vi "Get Serial Port Name.vi"(4 "Error In":errorcluster, 7 "PS Communication Port In":refnum<visa-resource-name>) -> (0 "Error Out":errorcluster, 2 "Serial Port Name":string, 3 "PS Communication Port Out":refnum<visa-resource-name>)   [LabVIEW 2024]
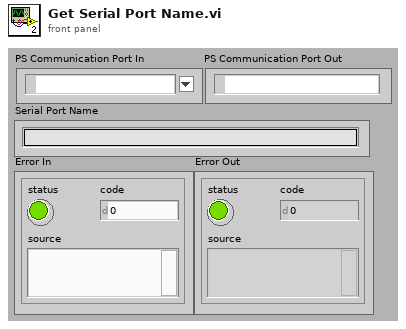
[diagram p1: front panel]
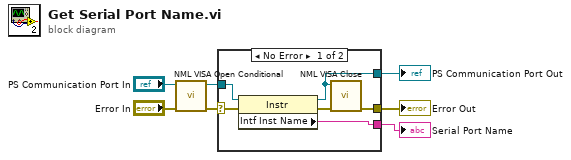
[diagram p0: block diagram]
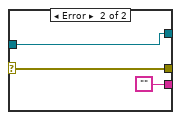
[diagram p2: hidden frame]
diagram:
  n1 = call "NML VISA Open Conditional.vi"("error in (no error)"="Error In", "VISA resource name"="PS Communication Port In") -> ("error out"=w5:errorcluster, "dup VISA Session"=w6:refnum<visa-resource-name>)  [unwired: 7 in, 1 out]
  n2 = case shown="No Error" w5 {
    selector: w5 -> [w10 w14]
    tunnel: [w13 w15] -> w7
    tunnel: [w9 ""] -> w4
    tunnel: w6 -> [w11 w15]
    tunnel: [w8 w14] -> w3
    frame No Error {
      n3 = property class="Instr"(reference=w11, error in=w10) -> (reference out=w13:refnum<visa-resource-name>, error out=w12:errorcluster, "Intf Inst Name"=w9:string)
      n4 = call "NML VISA Close.vi"("Error In"=w12, "VISA resource name"=w13) -> ("Error Out"=w8:errorcluster)  [unwired: 9 in]
    }
    frame Error {
    }
  }
  "PS Communication Port Out" <- w7
  "Serial Port Name" <- w4
  "Error Out" <- w3
